vi "Mode_driver.vi"(4 "error in (no error)":errorcluster, 6 "Action":enum16{"Launch", "Shutdown"}(ring)) -> (0 "error out":errorcluster, 3 "reference out (launch only)":refnum<vi>)   [LabVIEW 2015]
doc: "Provides an interface to the Primary Filter Manager. See the actions below.\n\nLaunch - launch the manager thread supplying references to the controls that the thread will update.\n\nHome - Home the primary filter\n\nMove - Move the primary filter to the position supplied by Filter#\n\nShutdown - Shutdown the fprimary filter manager"
uses:
  SystemUtil/Command.ctl
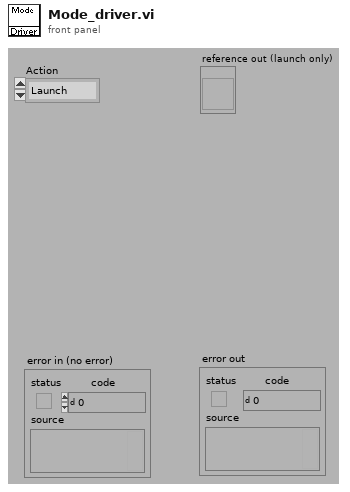
[diagram p1: front panel]
types:
  T1 = typedef "Command.ctl" = cluster{"Command":string, "Parameter":string}
  T2 = cluster{string, "type string":i16[], "data string":string}
  T3 = cluster{string, "type string":i16[], "data string":string}[]
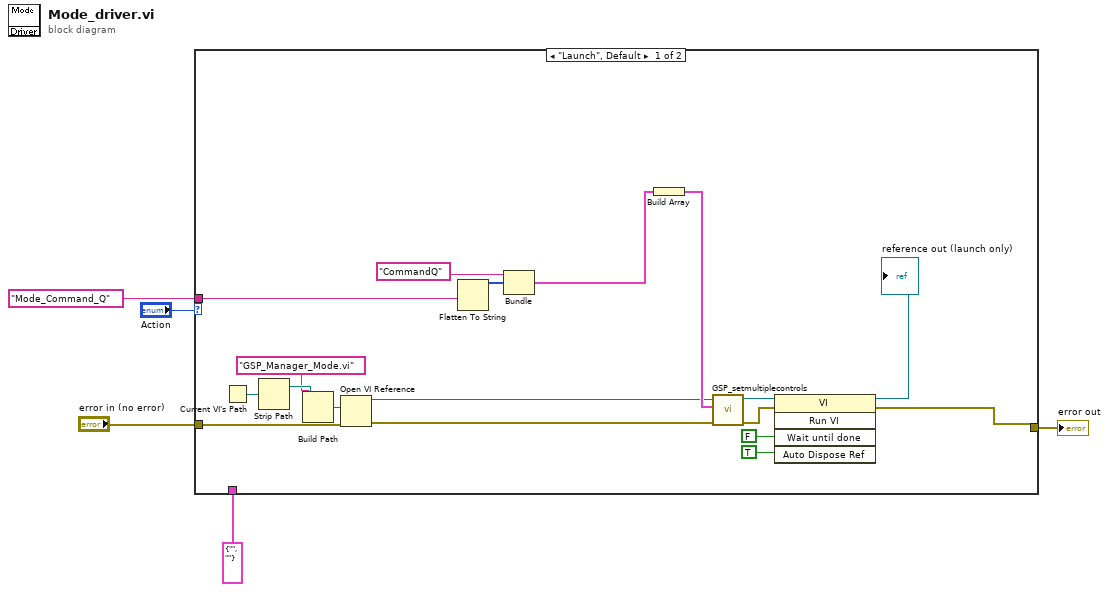
[diagram p0: block diagram]
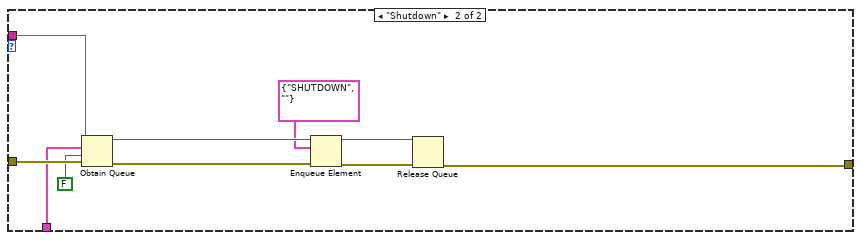
[diagram p2: hidden frame]
diagram:
  n1 = case shown="\"Launch\", Default" "Action" {
    tunnel: "error in (no error)" -> [w19 w34]
    tunnel: [w7 w25] -> w4
    tunnel: "Mode_Command_Q" -> [w8 w32]
    tunnel: T1 {"Command"="", "Parameter"=""} ("Command") -> [_ w29]
    frame "Launch", Default {
      n2 = Current VI's Path() -> (path=w12:path)
      n3 = Strip Path(path=w12) -> (stripped path=w10:path)  [unwired: 1 out]
      n4 = Build Path(base path=w10, name or relative path="GSP_Manager_Mode.vi" ("vi path")) -> (appended path=w11:path)
      n5 = Open VI Reference(vi path=w11, error in (no error)=w19) -> (vi reference=w17:refnum<vi>, error out=w18:errorcluster)  [unwired: 4 in]
      n6 = Flatten To String(anything=w8) -> (data string=w22:string, type string=w23:i16[])  [unwired: 3 in, 1 out]
      n7 = Bundle("CommandQ", "type string"=w23, "data string"=w22) -> (w21:T2)  [unwired: 1 in]
      n8 = Build Array(w21) -> (w20:T3)
      n9 = call "GSP_setmultiplecontrols.vi"("error in (no error)"=w18, "Control Infos"=w20, "reference"=w17) -> ("error out"=w15:errorcluster, "reference out"=w16:refnum<vi>)  [unwired: 3 in]
      n10 = invoke class="VI" method="Run VI"(reference=w16, error in=w15, "Wait until done"=FALSE, "Auto Dispose Ref"=TRUE) -> (reference out=→"reference out (launch only)":refnum<vi>, error out=w7:errorcluster)  [unwired: 1 in, 3 out]
    }
    frame "Shutdown" {
      n11 = Obtain Queue(name (unnamed)=w32, element data type=w29, create if not found? (T)=FALSE, error in (no error)=w34) -> (queue out=w31:refnum<queue>, error out=w33:errorcluster)  [unwired: 1 in, 1 out]
      n12 = Enqueue Element(queue=w31, element=T1 {"Command"="SHUTDOWN", "Parameter"=""}, error in (no error)=w33) -> (queue out=w27:refnum<queue>, error out=w26:errorcluster)  [unwired: 1 in, 1 out]
      n13 = Release Queue(queue=w27, error in (no error)=w26) -> (error out=w25:errorcluster)  [unwired: 1 in, 2 out]
    }
  }
  "error out" <- w4
